vi "Write Exec Reentrancy Type To VIs.vi"(11 "Array":T1[](array[typedef])) -> (0 "error out":errorcluster)   [LabVIEW 2022 SP3]
uses:
  TDs/FileProps.ctl
panel:
  out "Num Of Files":i32
  out "Idx":i32
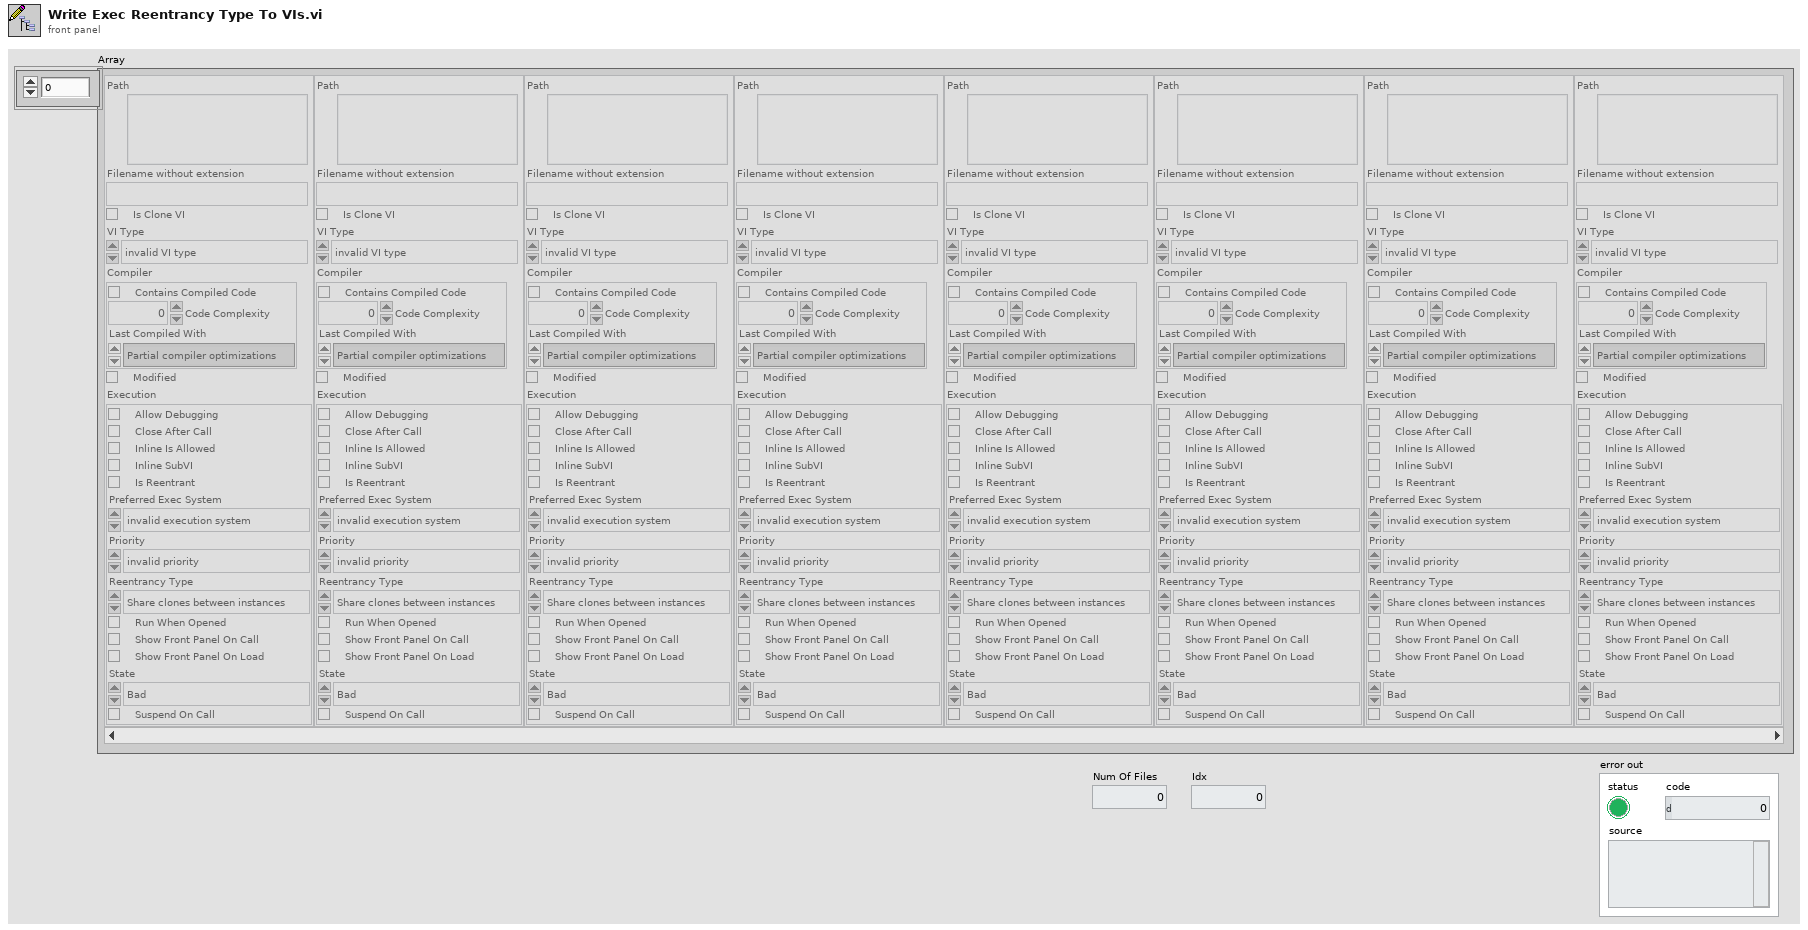
[diagram p1: front panel]
types:
  T1 = typedef "FileProps.ctl" = cluster{"Path":path, "Filename without extension":string, "Is Clone VI":bool, "VI Type":enum32{"invalid VI type", "Standard VI", "Control VI", "Global VI", "Polymorphic VI", "Configuration VI", "SubSystem", "Facade VI", "Method VI", "Statechart Diagram VI"}, "Compiler":cluster{"Contains Compiled Code":bool, "Code Complexity":sgl, "Last Compiled With":enum16{"Partial compiler optimizations", "Full compiler optimizations"}}, "Modified":bool, "Execution":cluster{"Allow Debugging":bool, "Close After Call":bool, "Inline Is Allowed":bool, "Inline SubVI":bool, "Is Reentrant":bool, "Preferred Exec System":enum32{"invalid execution system", "user interface", "standard", "instrument i/o", "data acquisition", "other 1", "other 2", "same as caller"}, "Priority":enum32{"invalid priority", "background priority", "normal priority", "above normal priority", "high priority", "time critical priority", "subroutine"}, "Reentrancy Type":enum16{"Share clones between instances", "Preallocate clone for each instance"}, "Run When Opened":bool, "Show Front Panel On Call":bool, "Show Front Panel On Load":bool, "State":enum32{"Bad", "Idle", "Run top level", "Running"}, "Suspend On Call":bool}}
  T2 = enum16{"Share clones between instances", "Preallocate clone for each instance"}
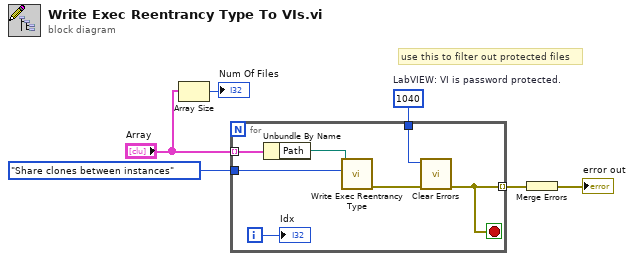
[diagram p0: block diagram]
diagram:
  w1 = 1040  # LabVIEW: VI is password protected.
  # "use this to filter out protected files"
  n1 = Array Size(array="Array") -> (size(s)=→"Num Of Files":i32)
  n2 = for {
    tunnel: "Array" -> [w13] mode=indexing
    tunnel: T2."Share clones between instances" ("Execution:Reentrancy Type") -> [w11]
    tunnel: [w8] -> w5 mode=indexing
    tunnel: w1 -> [w7]
    i -> [w10]
    stop <- w8 stop-if-true
    n3 = Unbundle By Name(w13) -> ("Path"=w12:path)
    n4 = call "Write Exec Reentrancy Type.vi"("Execution:Reentrancy Type"=w11, "file path"=w12) -> ("error out"=w9:errorcluster)  [unwired: 9 in]
    n5 = call <vilib>:"Clear Errors.vi"("error in (no error)"=w9, "specific error code to clear (0: all)"=w7) -> ("error out"=w8:errorcluster)  [unwired: 4 in, 1 out]
    "Idx" <- w10
  }
  n6 = Merge Errors(w5) -> (→"error out":errorcluster)
